vi "Read Data.vi"(8 "error in (no error)":errorcluster, 11 "bt_Blackboard in":refnum<class "bt_Blackboard.lvclass">) -> (0 "error out":errorcluster, 2 "Data":T1[](array[typedef]), 3 "bt_Blackboard out":refnum<class "bt_Blackboard.lvclass">)   [LabVIEW 2021, in "BT.lvlib" / "bt_Blackboard.lvclass"]
uses:
  bt_Blackboard.lvclass
  bt_Blackboard.lvclass/bt_Blackboard.ctl
  Support/Status Type.ctl
  Support/Data DVR Type.ctl
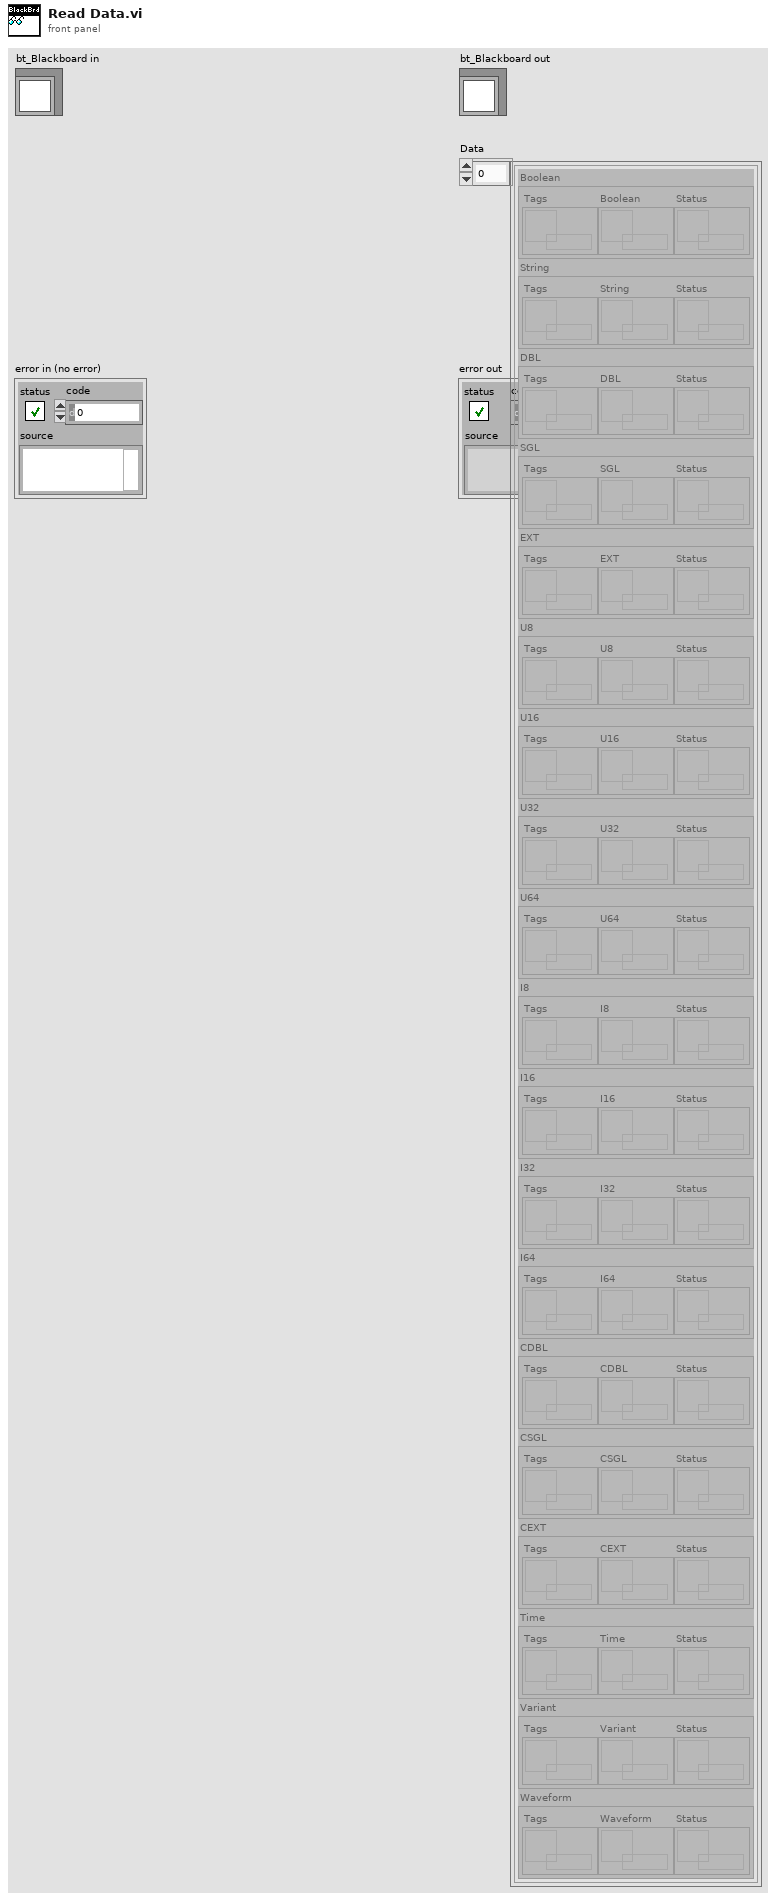
[diagram p1: front panel]
types:
  T1 = typedef "BT.lvlib/bt_Blackboard.lvclass/Data DVR Type.ctl" = cluster{"Boolean":cluster{"Tags":refnum<data-value>, "Boolean":refnum<data-value>, "Status":refnum<data-value>}, "String":cluster{"Tags":refnum<data-value>, "String":refnum<data-value>, "Status":refnum<data-value>}, "DBL":cluster{"Tags":refnum<data-value>, "DBL":refnum<data-value>, "Status":refnum<data-value>}, "SGL":cluster{"Tags":refnum<data-value>, "SGL":refnum<data-value>, "Status":refnum<data-value>}, "EXT":cluster{"Tags":refnum<data-value>, "EXT":refnum<data-value>, "Status":refnum<data-value>}, "U8":cluster{"Tags":refnum<data-value>, "U8":refnum<data-value>, "Status":refnum<data-value>}, "U16":cluster{"Tags":refnum<data-value>, "U16":refnum<data-value>, "Status":refnum<data-value>}, "U32":cluster{"Tags":refnum<data-value>, "U32":refnum<data-value>, "Status":refnum<data-value>}, "U64":cluster{"Tags":refnum<data-value>, "U64":refnum<data-value>, "Status":refnum<data-value>}, "I8":cluster{"Tags":refnum<data-value>, "I8":refnum<data-value>, "Status":refnum<data-value>}, "I16":cluster{"Tags":refnum<data-value>, "I16":refnum<data-value>, "Status":refnum<data-value>}, "I32":cluster{"Tags":refnum<data-value>, "I32":refnum<data-value>, "Status":refnum<data-value>}, "I64":cluster{"Tags":refnum<data-value>, "I64":refnum<data-value>, "Status":refnum<data-value>}, "CDBL":cluster{"Tags":refnum<data-value>, "CDBL":refnum<data-value>, "Status":refnum<data-value>}, "CSGL":cluster{"Tags":refnum<data-value>, "CSGL":refnum<data-value>, "Status":refnum<data-value>}, "CEXT":cluster{"Tags":refnum<data-value>, "CEXT":refnum<data-value>, "Status":refnum<data-value>}, "Time":cluster{"Tags":refnum<data-value>, "Time":refnum<data-value>, "Status":refnum<data-value>}, "Variant":cluster{"Tags":refnum<data-value>, "Variant":refnum<data-value>, "Status":refnum<data-value>}, "Waveform":cluster{"Tags":refnum<data-value>, "Waveform":refnum<data-value>, "Status":refnum<data-value>}}
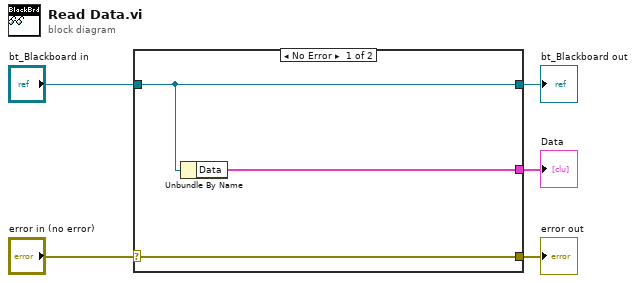
[diagram p0: block diagram]
diagram:
  n1 = case shown="No Error" "error in (no error)" {
    selector: "error in (no error)" -> [w8 w9]
    tunnel: [w8 w9] -> w4
    tunnel: [w7 w10] -> w2
    tunnel: "bt_Blackboard in" -> [w7 w10]
    tunnel: [w6 _] -> w1
    frame No Error {
      n2 = Unbundle By Name(w7) -> ("Data"=w6:T1[])
    }
    frame Error {
    }
  }
  "error out" <- w4
  "bt_Blackboard out" <- w2
  "Data" <- w1
